vi "Set battery alert status.vi"(7 "Error In":errorcluster, 8 "Alert status":bool, 9 "MAC address":string) -> (0 "Error Out":errorcluster)   [LabVIEW 2016]
uses:
  <vilib>/Utility/file.llb/Read Delimited Spreadsheet (string).vi
  <vilib>/Utility/file.llb/Write Delimited Spreadsheet (string).vi
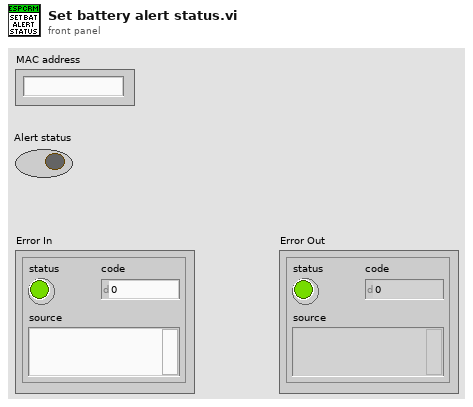
[diagram p1: front panel]
types:
  T1 = enum16{"open", "replace", "create", "open or create", "replace or create", "replace or create with confirmation"}
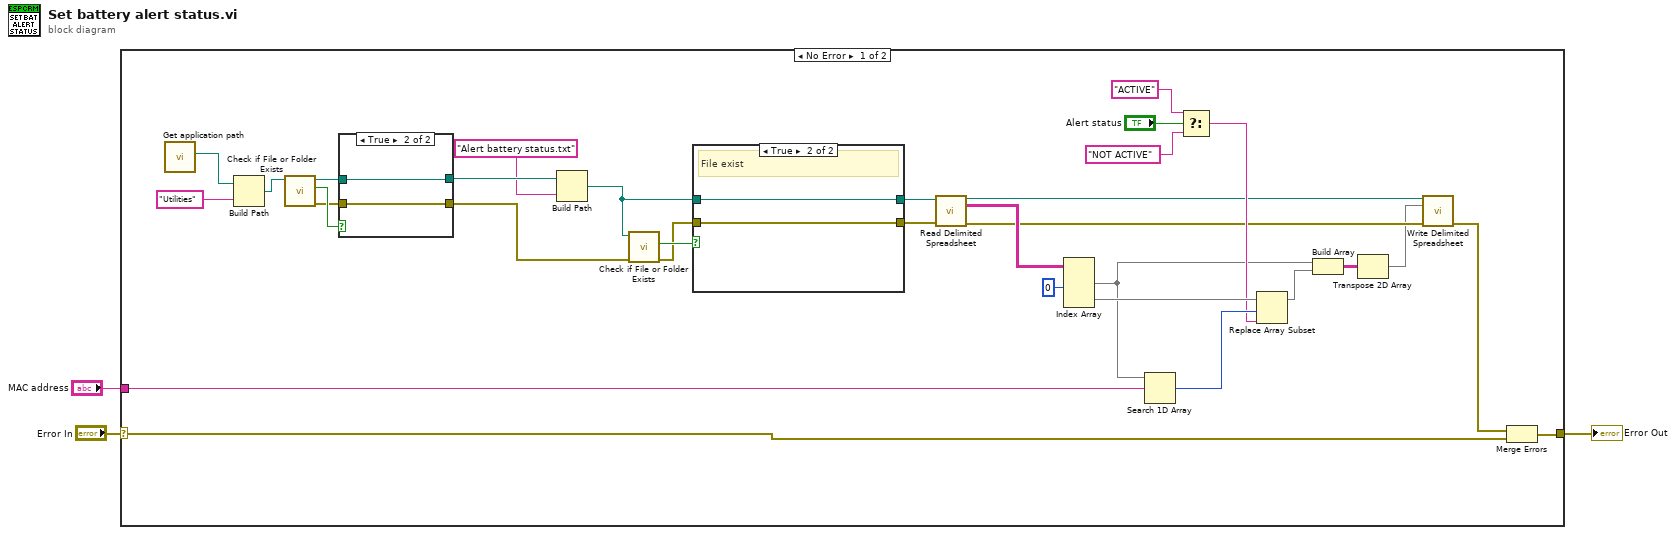
[diagram p0: block diagram]
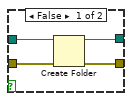
[diagram p2: hidden frame]
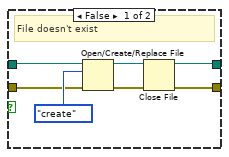
[diagram p3: hidden frame]
diagram:
  n1 = case shown="No Error" "Error In" {
    selector: "Error In" -> [w8 w51]
    tunnel: "MAC address" -> [w20 _]
    tunnel: [w10 w51] -> w1
    frame No Error {
      n2 = call "Get application path.vi"() -> ("Application path"=w26:path)  [unwired: 11 in]
      n3 = Build Path(base path=w26, name or relative path="Utilities") -> (appended path=w28:path)
      n4 = call <vilib>:"Check if File or Folder Exists.vi"("path"=w28) -> ("error out"=w32:errorcluster, "file or folder exists?"=w33:bool, "dup path"=w31:path)  [unwired: 8 in]
      n5 = case shown="True" w33 {
        tunnel: w32 -> [w39 w40]
        tunnel: w31 -> [w38 w41]
        tunnel: [w37 w41] -> w30
        tunnel: [w36 w40] -> w25
        frame False {
          n6 = Create Folder(path (use dialog)=w38, error in=w39) -> (created path=w37:path, error out=w36:errorcluster)  [unwired: 1 in, 1 out]
        }
        frame True {
        }
      }
      n7 = Build Path(base path=w30, name or relative path="Alert battery status.txt") -> (appended path=w34:path)
      n8 = call <vilib>:"Check if File or Folder Exists.vi"("error in (no error)"=w25, "path"=w34) -> ("error out"=w24:errorcluster, "file or folder exists?"=w35:bool)  [unwired: 7 in, 1 out]
      n9 = case shown="True" w35 {
        tunnel: [w45 w50] -> w21
        tunnel: w34 -> [w44 w50]
        tunnel: w24 -> [w43 w49]
        tunnel: [w42 w49] -> w11
        frame False {
          # "File doesn't exist"
          n10 = Open/Create/Replace File(file path (use dialog)=w44, error in=w43, operation (0:open)=T1."create") -> (refnum out=w46:refnum<file>, error out=w47:errorcluster)  [unwired: 3 in, 1 out]
          n11 = Close File(refnum=w46, error in=w47) -> (path=w45:path, error out=w42:errorcluster)
        }
        frame True {
          # "File exist"
        }
      }
      n12 = call-poly <vilib>:"Read Delimited Spreadsheet.vi"("file path (dialog if empty)"=w21, "error in (no error)"=w11) -> ("new file path (Not A Path if cancelled)"=w13:path, "all rows"=w23:string[][], "error out"=w12:errorcluster)  [unwired: 8 in, 3 out]
      n13 = Index Array(array=w23, index (col) #1=0 ("disabled index (col)")) -> (element #1=w6:string[], element #2=w16:string[])  [unwired: 3 in]
      n14 = Search 1D Array(1D array=w6, element=w20) -> (index of element=w15:i32)  [unwired: 1 in]
      n15 = Select(t="ACTIVE", s="Alert status", f="NOT ACTIVE") -> (s? t:f=w14:string)
      n16 = Replace Array Subset(array=w16, new element=w14, index=w15) -> (w7:string[])
      n17 = Build Array(w6, w7) -> (w5:string[][])
      n18 = Transpose 2D Array(2D array=w5) -> (transposed array=w4:string[][])
      n19 = call-poly <vilib>:"Write Delimited Spreadsheet.vi"("file path (dialog if empty)"=w13, "2D data"=w4, "error in (no error)"=w12) -> ("error out"=w9:errorcluster)  [unwired: 11 in, 1 out]
      n20 = Merge Errors(w9, w8) -> (w10:errorcluster)
    }
    frame Error {
    }
  }
  "Error Out" <- w1
